vi "Laudatest.vi"() -> ()   [LabVIEW 2017]
uses:
  BERTTA.dll
panel:
  in  "set_temp":dbl
  in  "port":i32
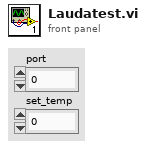
[diagram p1: front panel]
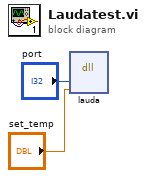
[diagram p0: block diagram]
diagram:
  n1 = dll-call lib="C:/Users/p3cn/OneDrive - Kemira Oyj/Documents/GitHub/Bertta/BERTTA/x64/Debug/BERTTA.dll" fn="lauda"("port"="port", "set_temp"="set_temp") -> ()  [unwired: 6 in, 2 out]
